vi "Functionalie NS.vi"(9 "Molecle Area with Gap":dbl, 10 "# of CNTs in 1 NS":dbl, 11 "Surface Area of 1 CNT":dbl) -> (1 "Total Functionalized Molecules on NS":dbl, 2 "Concentration on 1 NS (Moles/m3)":ext[unit], 3 "Concentration,  M":ext[unit], 4 "No of Molecules on 1 CNT Functionalized":dbl)   [LabVIEW 2020]
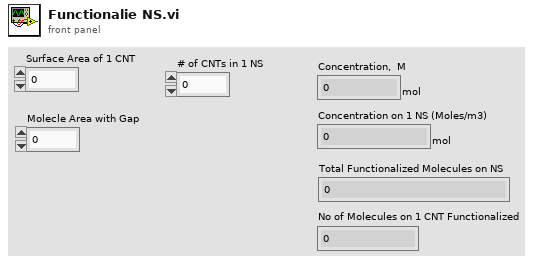
[diagram p1: front panel]
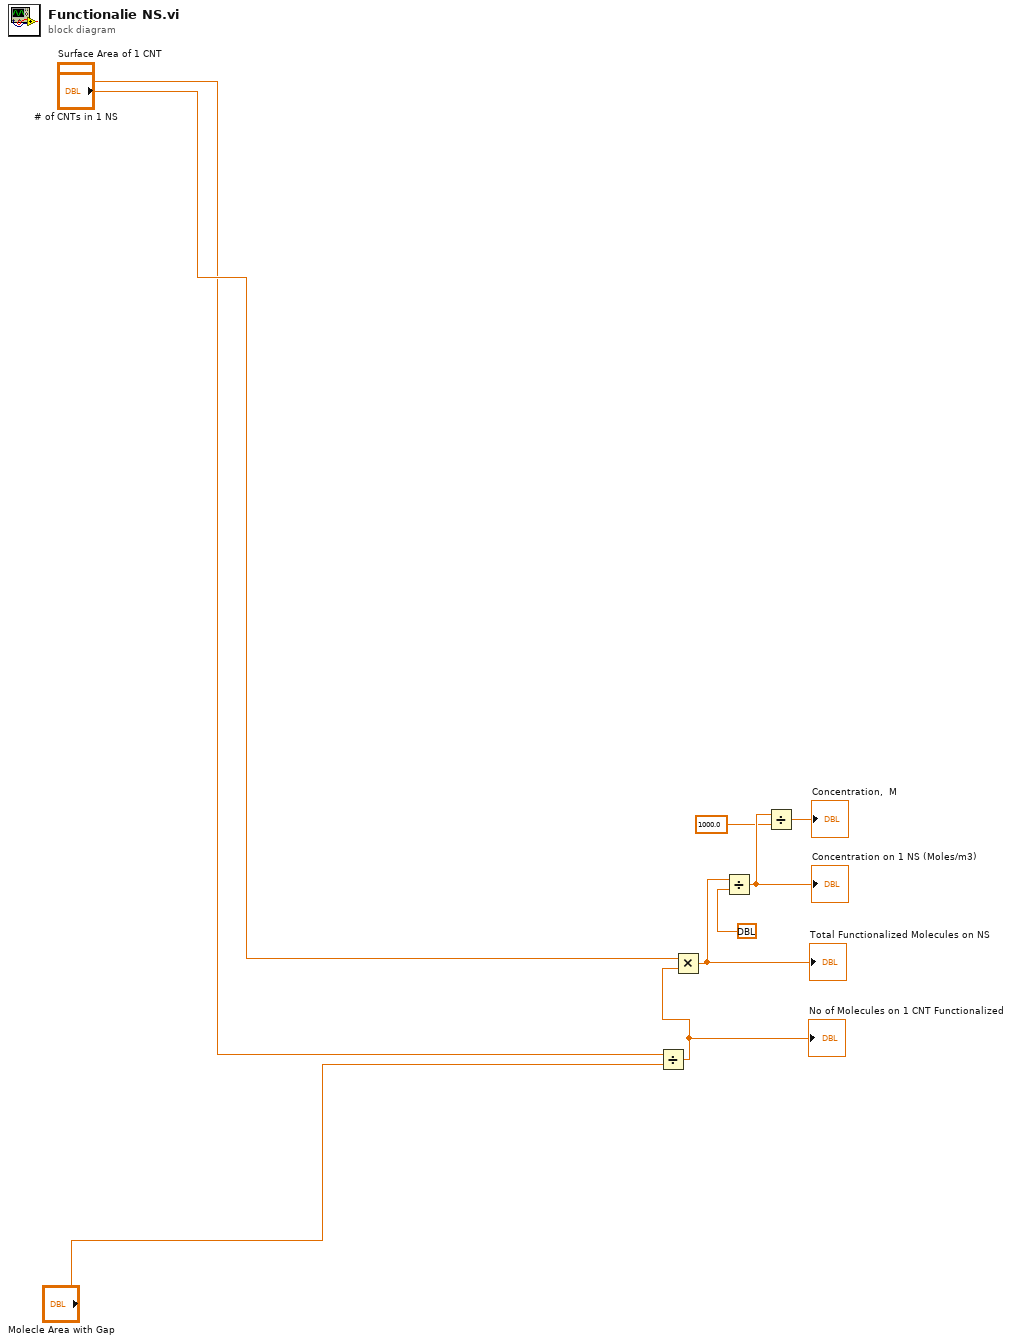
[diagram p0: block diagram]
diagram:
  n1 = Divide(x="Surface Area of 1 CNT", y="Molecle Area with Gap") -> (x/y=w1:dbl)
  "No of Molecules on 1 CNT Functionalized" <- w1
  n2 = Multiply(x="# of CNTs in 1 NS", y=w1) -> (x*y=w3:dbl)
  "Total Functionalized Molecules on NS" <- w3
  n3 = Divide(x=w3, y=ext[unit] 6.0221408569999999998e+23) -> (x/y=w5:ext[unit])
  "Concentration on 1 NS (Moles/m3)" <- w5
  n4 = Divide(x=w5, y=1000.0) -> (x/y=→"Concentration,  M":ext[unit])
